vi "skip.vi"(8 "error in (no error)":errorcluster, 10 "skipMessage":string, 11 "TestSuite in":refnum<class "TestSuite.lvclass">) -> (0 "error out":errorcluster, 3 "TestSuite out":refnum<class "TestSuite.lvclass">)   [LabVIEW 2013, in "TestSuite.lvclass"]
doc: "Causes TestSuite to be skipped (and not actually run)."
uses:
  TestSuite.lvclass
  TestSuite.lvclass/TestSuite.ctl
panel:
  # "JKI VI Tester for LabVIEW\nhttp://jkisoft.com/vi-tester\nCopyright (C) 2007-2009, JKI <info@jkisoft.com>\nALL RIGHTS RESERVED"
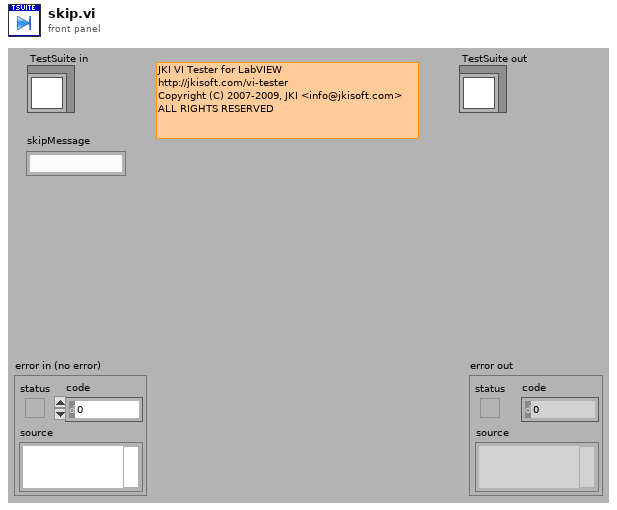
[diagram p1: front panel]
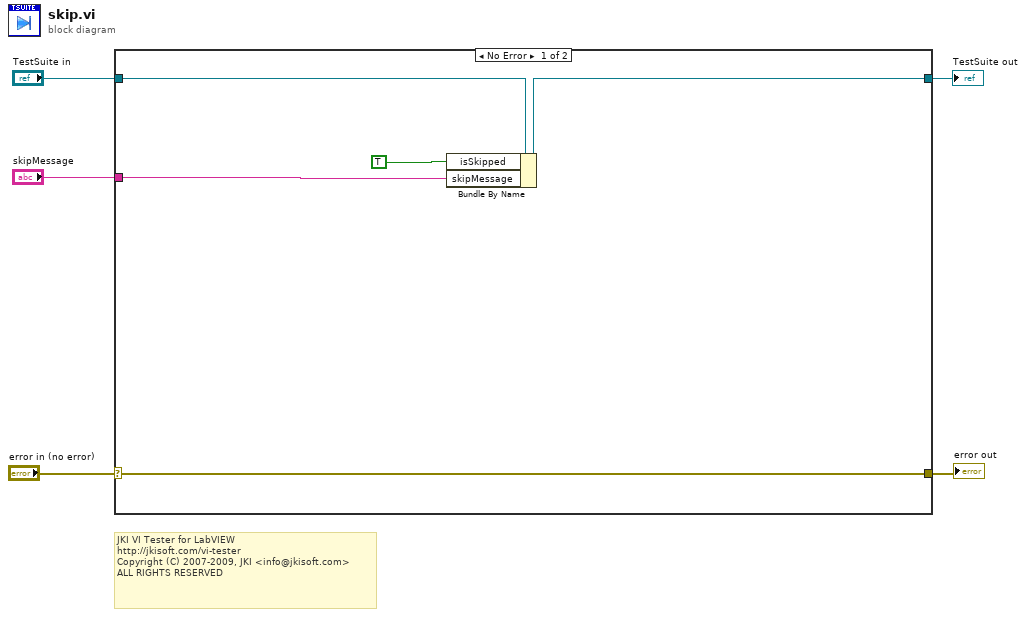
[diagram p0: block diagram]
diagram:
  # "JKI VI Tester for LabVIEW\nhttp://jkisoft.com/vi-tester\nCopyright (C) 2007-2009, JKI <info@jkisoft.com>\nALL RIGHTS RESERVED"
  n1 = case shown="No Error" "error in (no error)" {
    selector: "error in (no error)" -> [w10 w12]
    tunnel: [w10 w12] -> w4
    tunnel: [w8 w11] -> w2
    tunnel: "TestSuite in" -> [w9 w11]
    tunnel: "skipMessage" -> [w6 _]
    frame No Error {
      n2 = Bundle By Name(cluster=w9, "isSkipped"=TRUE, "skipMessage"=w6) -> (w8:refnum<class "TestSuite.lvclass">)
    }
    frame Error {
    }
  }
  "error out" <- w4
  "TestSuite out" <- w2
